vi "getdrive joystick.vi"() -> (2 "drive joystick buttons":bool[](array[boolean]), 3 "drive joystick values":dbl[](array[numeric]))   [LabVIEW 2019]
doc: "Gets the Drive Joystick"
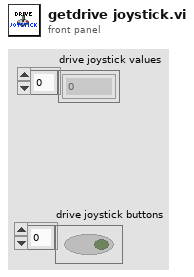
[diagram p1: front panel]
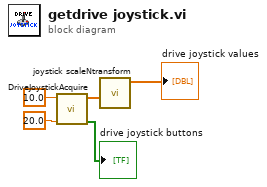
[diagram p0: block diagram]
diagram:
  n1 = call "DriveJoystickAcquire.vi"("Rotation Joystick Deadband %"=20.0, "XY Joystick Deadband %"=10.0) -> ("Drive Joystick Buttons"=→"drive joystick buttons":bool[], "Drive Joystick Values"=w3:dbl[])  [unwired: 7 in, 1 out]
  n2 = call "joystick scaleNtransform.vi"("joystick values"=w3) -> ("Transformed joystick values"=→"drive joystick values":dbl[])  [unwired: 10 in]
